vi "Pre Launch Init.vi"(11 "UI Status in":refnum<class "UI Status.lvclass">) -> (0 "error out":errorcluster, 3 "UI Status out":refnum<class "UI Status.lvclass">)   [LabVIEW 2020, in "UI Status.lvlib" / "UI Status.lvclass"]
doc: "(<B>Filename</B>: Actor Framework.lvlib:Actor.lvclass:Pre Launch Init.vi)\n\nDefines behavior that occurs after the Launch Nested Actor method is invoked but before the actor's Actor Core method begins running.\n\nBy default, this method does nothing. A descendant class may override it to define behavior."
uses:
  UI Status.lvclass
  UI Status.lvclass/UI Status.ctl
  <vilib>/ActorFramework/Actor/Actor.lvclass
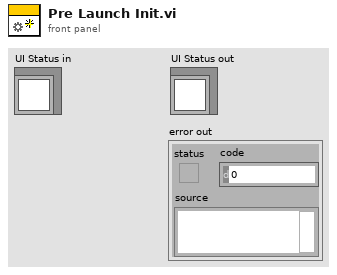
[diagram p1: front panel]
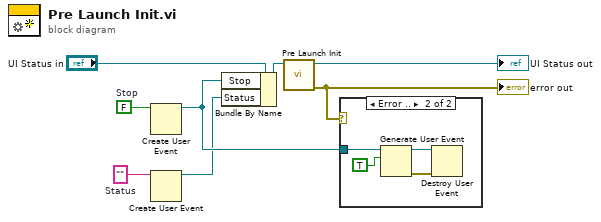
[diagram p0: block diagram]
diagram:
  w2 = ""  # Status
  w7 = FALSE  # Stop
  n1 = Create User Event(user event datatype=w7) -> (user event=w3:refnum<user-event>)  [unwired: 1 in, 1 out]
  n2 = Create User Event(user event datatype=w2) -> (user event=w1:refnum<user-event>)  [unwired: 1 in, 1 out]
  n3 = Bundle By Name(cluster="UI Status in", "Stop"=w3, "Status"=w1) -> (w5:refnum<class "UI Status.lvclass">)
  n4 = call-parent "Pre Launch Init.vi"("Actor in"=w5) -> ("error out"=w4:errorcluster, "Actor out"=→"UI Status out":refnum<class "UI Status.lvclass">)  [unwired: 9 in]
  "error out" <- w4
  n5 = case shown="Error .." w4 {
    tunnel: w3 -> [_ w12]
    frame No Error {
    }
    frame Error {
      n6 = Generate User Event(user event=w12, event data cluster=TRUE ("event data")) -> (user event out=w9:refnum<user-event>, error out=w10:errorcluster)  [unwired: 2 in]
      n7 = Destroy User Event(user event=w9, error in=w10) -> ()  [unwired: 1 out]
    }
  }
